vi "JsonString To VariantStringAttrs.vi"(8 "error in (no error)":errorcluster, 11 "Json":string) -> (0 "error out":errorcluster, 3 "Variant":variant)   [LabVIEW 2019, in "lv-apt-json-file.lvlib"]
uses:
  lv-apt-json-file.lvlib
  <vilib>/addons/_JKI.lib/Serialization/JSON/JKI JSON Serialization.lvlib
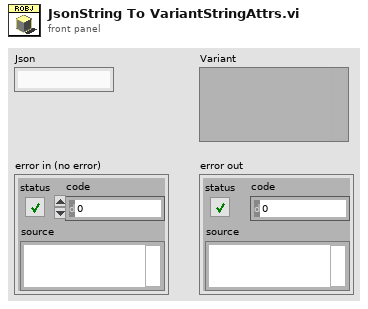
[diagram p1: front panel]
types:
  T1 = typedef "Type Descriptor Enumeration__ogtk.ctl" = enum8{"<Null>", "I8", "I16", "I32", "I64", "U8", "U16", "U32", "U64", "SGL", "DBL", "EXT", "CSG", "CDB", "CXT", "0x0F", "0x10", "0x11", "0x12", "0x13", "0x14", "Enum U8", "Enum U16", "Enum U32", "Enum U64", "SGL PQ", "DBL PQ", "EXT PQ", "CSG PQ", "CDB PQ", "CXT PQ", "0x1F", "0x20", "Boolean", "0x22", "0x23", "0x24", "0x25", "0x26", "0x27", "0x28", "0x29", "0x2A", "0x2B", "0x2C", "0x2D", "0x2E", "0x2F", "String", "0x31", "Path", "Pict", "0x34", "0x35", "0x36", "DAQ", "0x38", "0x39", "0x3A", "0x3B", "0x3C", "0x3D", "0x3E", "0x3F", "Array", "0x41", "0x42", "0x43", "0x44", "0x45", "0x46", "0x47", "0x48", "0x49", "0x4A", "0x4B", "0x4C", "0x4D", "0x4E", "0x4F", "Cluster", "0x51", "0x52", "Variant", "Waveform", "0x55", "0x56", "0x57", "0x58", "0x59", "0x5A", "0x5B", "0x5C", "0x5D", "0x5E", "0x5F", "0x60", "0x61", "0x62", "0x63", "0x64", "0x65", "0x66", "0x67", "0x68", "0x69", "0x6A", "0x6B", "0x6C", "0x6D", "0x6E", "0x6F", "Refnum"}
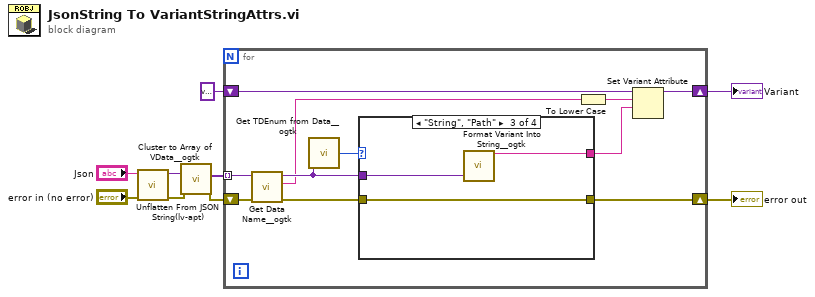
[diagram p0: block diagram]
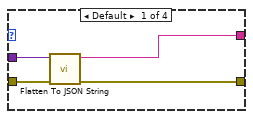
[diagram p2: hidden frame]
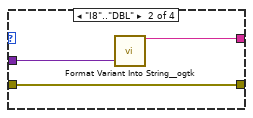
[diagram p3: hidden frame]
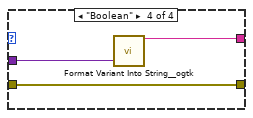
[diagram p4: hidden frame]
diagram:
  n1 = call "Unflatten From JSON String(lv-apt).vi"("error in (no error)"="error in (no error)", "JSON String"="Json") -> ("error out"=w1:errorcluster, "Variant"=w2:variant)  [unwired: 8 in]
  n2 = call <userlib>:"Cluster to Array of VData__ogtk.vi"("error in (no error)"=w1, "Cluster"=w2) -> ("error out"=w4:errorcluster, "Array of VData"=w3:variant[])  [unwired: 8 in]
  n3 = for {
    tunnel: w3 -> [w20] mode=indexing
    shift-right: [w15] -> w5
    shift-left: variant -> [w14]
    shift-right: [w10] -> w8
    shift-left: w4 -> [w16]
    n4 = call <userlib>:"Get Data Name__ogtk.vi"("error in (no error)"=w16, "Data"=w20) -> ("error out"=w18:errorcluster, "Data Name"=w13:string, "Data dup"=w17:variant)  [unwired: 7 in]
    n5 = call <userlib>:"Get TDEnum from Data__ogtk.vi"("Data"=w17) -> ("Type Descriptor Enumeration"=w19:T1)  [unwired: 4 in]
    n6 = case shown="\"String\", \"Path\"" w19 {
      tunnel: w18 -> [w23 w25 w28 w31]
      tunnel: w17 -> [w24 w27 w30 w33]
      tunnel: [w22 w26 w29 w32] -> w12
      tunnel: [w21 w25 w28 w31] -> w10
      frame Default {
        n7 = call <vilib>:"Flatten To JSON String.vi"("error in (no error)"=w23, "Variant"=w24) -> ("error out"=w21:errorcluster, "JSON String"=w22:string)  [unwired: 8 in]
      }
      frame "I8".."DBL" {
        n8 = call <userlib>:"Format Variant Into String__ogtk.vi"("Variant"=w27) -> ("Output String"=w26:string)  [unwired: 13 in, 1 out]
      }
      frame "String", "Path" {
        n9 = call <userlib>:"Format Variant Into String__ogtk.vi"("Variant"=w30) -> ("Output String"=w29:string)  [unwired: 13 in, 1 out]
      }
      frame "Boolean" {
        n10 = call <userlib>:"Format Variant Into String__ogtk.vi"("Variant"=w33) -> ("Output String"=w32:string)  [unwired: 13 in, 1 out]
      }
    }
    n11 = To Lower Case(string=w13) -> (all lower case string=w11:string)
    n12 = Set Variant Attribute(Variant=w14, name=w11, value=w12) -> (Variant out=w15:variant)  [unwired: 1 in, 2 out]
  }
  "error out" <- w8
  "Variant" <- w5
